vi "Error Manager.vi"(5 "Error In":errorcluster) -> (19 "Error Out":errorcluster)   [LabVIEW 2015]
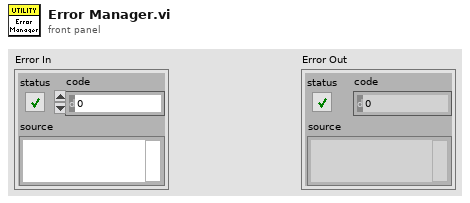
[diagram p1: front panel]
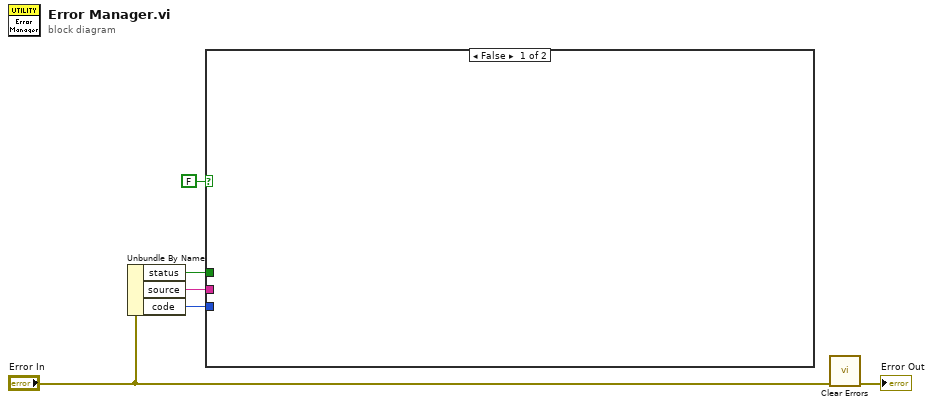
[diagram p0: block diagram]
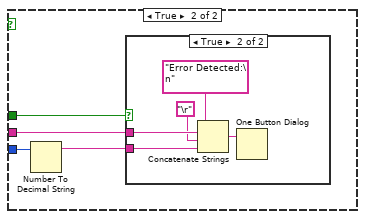
[diagram p2: hidden frame]
diagram:
  n1 = Unbundle By Name("Error In") -> ("status"=w1:bool, "source"=w2:string, "code"=w3:i32)
  n2 = case shown="False" FALSE {
    tunnel: w3 -> [_ w10]
    tunnel: w2 -> [_ w9]
    tunnel: w1 -> [_ w7]
    frame False {
    }
    frame True {
      n3 = Number To Decimal String(number=w10) -> (decimal integer string=w8:string)  [unwired: 1 in]
      n4 = case shown="True" w7 {
        tunnel: w9 -> [_ w13]
        tunnel: w8 -> [_ w11]
        frame False {
        }
        frame True {
          n5 = Concatenate Strings("Error Detected:\n" ("string"), w13, "\r", w11) -> (w15:string)
          n6 = One Button Dialog(message=w15) -> ()  [unwired: 1 in, 1 out]
        }
      }
    }
  }
  n7 = call <vilib>:"Clear Errors.vi"("error in (no error)"="Error In") -> ("error out"=→"Error Out":errorcluster)  [unwired: 5 in, 1 out]
